vi "Lifter Button.vi"(9 "Button":dbl, 10 "Axis":dbl) -> (2 "Output":dbl)   [LabVIEW 2014]
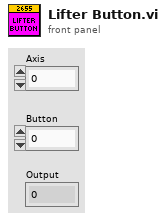
[diagram p1: front panel]
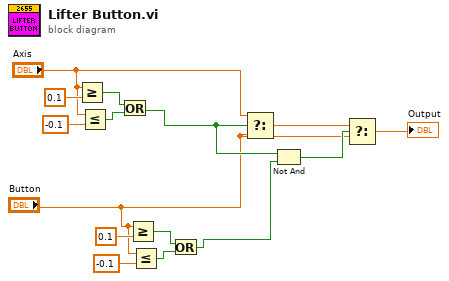
[diagram p0: block diagram]
diagram:
  n1 = Greater Or Equal?(x="Axis", y=0.1) -> (x >= y?=w7:bool)
  n2 = Less Or Equal?(x="Axis", y=-0.1) -> (x <= y?=w9:bool)
  n3 = Or(x=w7, y=w9) -> (x .or. y?=w8:bool)
  n4 = Greater Or Equal?(x="Button", y=0.1) -> (x >= y?=w3:bool)
  n5 = Less Or Equal?(x="Button", y=-0.1) -> (x <= y?=w4:bool)
  n6 = Or(x=w3, y=w4) -> (x .or. y?=w2:bool)
  n7 = Select(t="Axis", s=w8, f="Button") -> (s? t:f=w13:dbl)
  n8 = Not And(1:w2, 2:w8) -> (0:w14:bool)
  n9 = Select(t=w13, s=w14, f="Button") -> (s? t:f=→"Output":dbl)
